vi "Log Broadcast.vi"(8 "error in":errorcluster, 10 "Broadcast Name":string, 11 "Message Data In":variant) -> (0 "error out":errorcluster)   [LabVIEW 2015, in "Generic Module Library.lvlib" / "Template G_Module.lvlib"]
uses:
  Template G_Module.lvlib
  Module Class/Rename.lvclass
panel:
  out "Message Data Out":variant
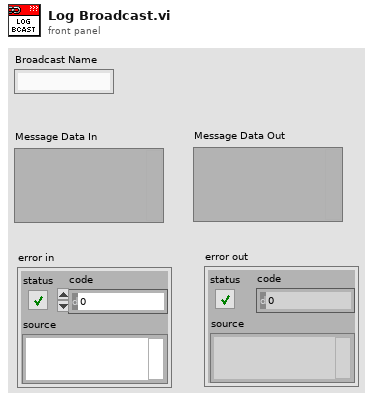
[diagram p1: front panel]
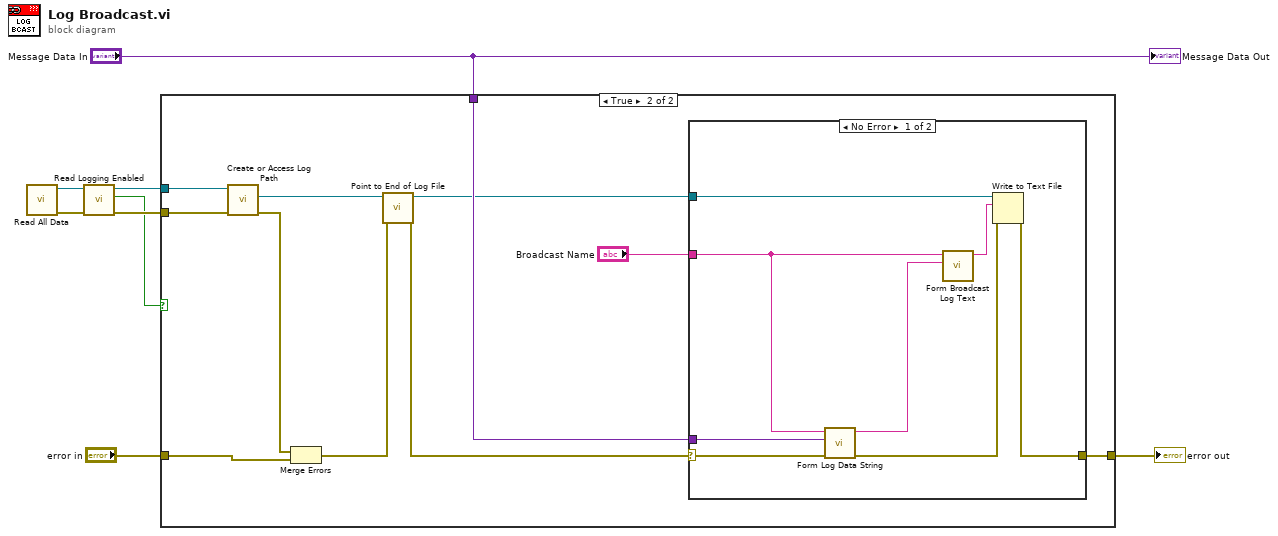
[diagram p0: block diagram]
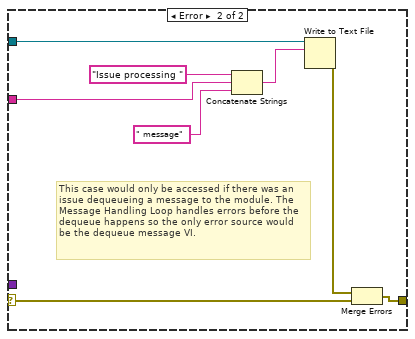
[diagram p3: hidden frame]
diagram:
  n1 = call "Read All Data.vi"() -> ("error out"=w3:errorcluster, "Data Out"=w5:refnum<class "Rename.lvclass">)  [unwired: 10 in]
  n2 = call-dynamic "Read Logging Enabled.vi"("error in (no error)"=w3, "Rename in"=w5) -> ("error out"=w2:errorcluster, "Logging Enabled"=w1:bool, "Rename out"=w4:refnum<class "Rename.lvclass">)  [unwired: 7 in]
  n3 = case shown="True" w1 {
    tunnel: [w9 w20] -> w8
    tunnel: "error in" -> [w9 w19]
    tunnel: "Message Data In" -> [_ w17]
    tunnel: w4 -> [_ w11]
    tunnel: w2 -> [_ w10]
    frame False {
    }
    frame True {
      n4 = call "Create or Access Log Path.vi"("error in"=w10, "Module Data In"=w11) -> ("error out"=w18:errorcluster, "Log Refnum Out"=w16:refnum<file>)  [unwired: 6 in, 2 out]
      n5 = Merge Errors(w18, w19) -> (w14:errorcluster)
      n6 = call "Point to End of Log File.vi"("error in (no error)"=w14, "Byte Stream File in"=w16) -> ("error out"=w13:errorcluster, "Byte Stream File out"=w15:refnum<file>)  [unwired: 8 in]
      n7 = case shown="No Error" w13 {
        selector: w13 -> [w24 w32]
        tunnel: w15 -> [w25 w36]
        tunnel: [w28 w34] -> w20
        tunnel: "Broadcast Name" -> [w27 w29]
        tunnel: w17 -> [w26 _]
        frame No Error {
          n8 = call "Form Log Data String.vi"("error in (no error)"=w24, "Message Data In"=w26, "Log Text"=w27) -> ("error out"=w22:errorcluster, "Log Data String"=w21:string)  [unwired: 7 in]
          n9 = call "Form Broadcast Log Text.vi"("Data String Input"=w21, "Broadcast"=w27) -> ("String to Write"=w23:string)  [unwired: 9 in]
          n10 = Write to Text File(file (use dialog)=w25, text=w23, error in=w22) -> (error out=w28:errorcluster)  [unwired: 1 in, 2 out]
        }
        frame Error {
          # "This case would only be accessed if there was an issue dequeueing a message to the module. The Message Handling Loop handles errors before the dequeue happens so the only error source would be the dequeue message VI."
          n11 = Concatenate Strings("Issue processing " ("string"), w29, " message" ("string")) -> (w35:string)
          n12 = Write to Text File(file (use dialog)=w36, text=w35) -> (error out=w33:errorcluster)  [unwired: 2 in, 2 out]
          n13 = Merge Errors(w33, w32) -> (w34:errorcluster)
        }
      }
    }
  }
  "error out" <- w8
  "Message Data Out" <- "Message Data In"
